vi "Initialize.vi"(8 "error in (no error)":errorcluster, 9 "ID Query":bool, 10 "Reset":bool, 11 "National Instrument USB-6501 in":refnum<class "National Instrument USB-6501.lvclass">) -> (0 "error out":errorcluster, 2 "VISA resource name":refnum<visa-resource-name>, 3 "National Instrument USB-6501 out":refnum<class "National Instrument USB-6501.lvclass">)   [LabVIEW 2014, in "Generic Data Acquisition.lvlib" / "National Instrument USB-6501.lvlib" / "National Instrument USB-6501.lvclass"]
uses:
  National Instrument USB-6501.lvclass
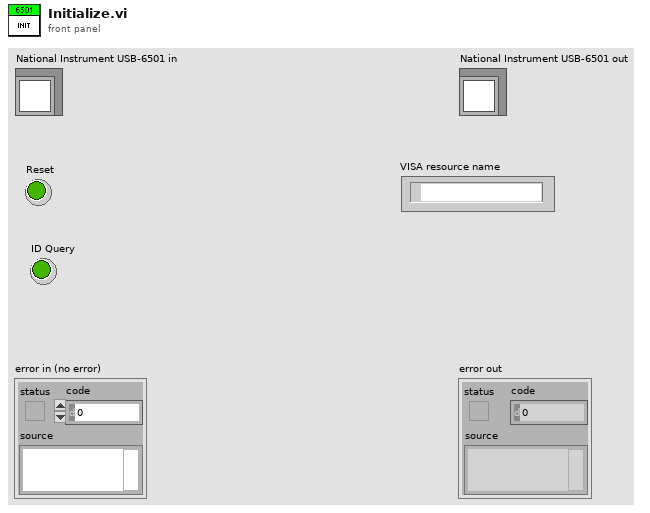
[diagram p1: front panel]
types:
  T1 = typedef "Data Acquisition Channel Settings.ctl" = cluster{"Function":enum16{"Digital Input", "Digital Output"}, "Port":i8, "Line":i8, "Name":string}
  T2 = cluster{"Function":enum16{"Digital Input", "Digital Output"}, "DAQmx Global Channel":refnum<k21>}
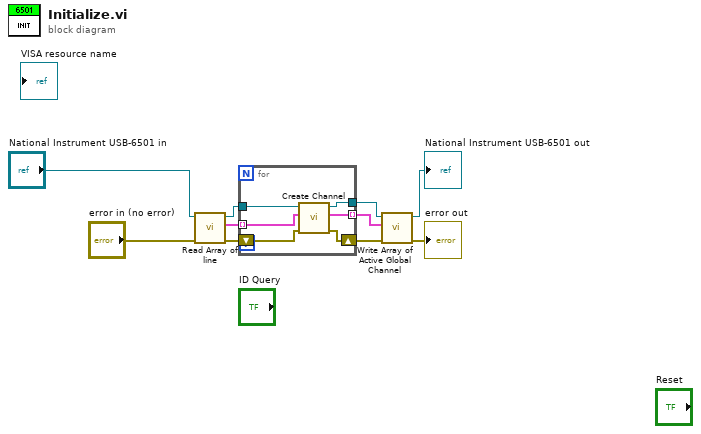
[diagram p0: block diagram]
diagram:
  n1 = call-dynamic "Read Array of line.vi"("error in (no error)"="error in (no error)", "National Instrument USB-6501 in"="National Instrument USB-6501 in") -> ("error out"=w1:errorcluster, "Array of line"=w8:T1[], "National Instrument USB-6501 out"=w7:refnum<class "National Instrument USB-6501.lvclass">)  [unwired: 7 in]
  n2 = for {
    tunnel: w8 -> [w11] mode=indexing
    tunnel: w7 -> [w16]
    tunnel: [w15] -> w6
    shift-right: [w13] -> w2
    shift-left: w1 -> [w14]
    tunnel: [w12] -> w5 mode=indexing
    n3 = call-dynamic "Create Channel.vi"("error in (no error)"=w14, "I/O"=w11, "National Instrument USB-6501 in"=w16) -> ("error out"=w13:errorcluster, "Cluster"=w12:T2, "National Instrument USB-6501 out"=w15:refnum<class "National Instrument USB-6501.lvclass">)  [unwired: 5 in, 1 out]
  }
  n4 = call-dynamic "Write Array of Active Global Channel.vi"("error in (no error)"=w2, "Array of Active Global Channel"=w5, "National Instrument USB-6501 in"=w6) -> ("error out"=→"error out":errorcluster, "National Instrument USB-6501 out"=→"National Instrument USB-6501 out":refnum<class "National Instrument USB-6501.lvclass">)  [unwired: 7 in]
